vi "Read Data.vi"(8 "error in (no error)":errorcluster, 11 "Serial Config":T1={"串口选择"="", "通讯速率"=9600, "超时时间"=10000, "数据位长"=8, "奇偶校验"=enum."None", "停止位长"=10, "握手控制"=0, "字符结束"=TRUE, "结束字符"=10} {"结束字符" format="%.0x"; "握手控制" items=["None", "XON/XOFF", "RTS/CTS", "XON/XOFF & RTS/CTS", "DTR/DSR", "XON/XOFF & DTR/DSR"]; "停止位长" items=["1.0"=10, "1.5"=15, "2.0"=20]; "数据位长" min=5 max=8 step=1}) -> (0 "error out":errorcluster, 2 "状态信息":string, 3 "返回值":dbl)   [LabVIEW 2010, in "CenterOne.lvlib"]
doc: "Use this template to build a VI to use as a subVI."
uses:
  CenterOne.lvlib
  Serial Config.ctl
  <vilib>/Instr/_visa.llb/VISA Configure Serial Port (Instr).vi
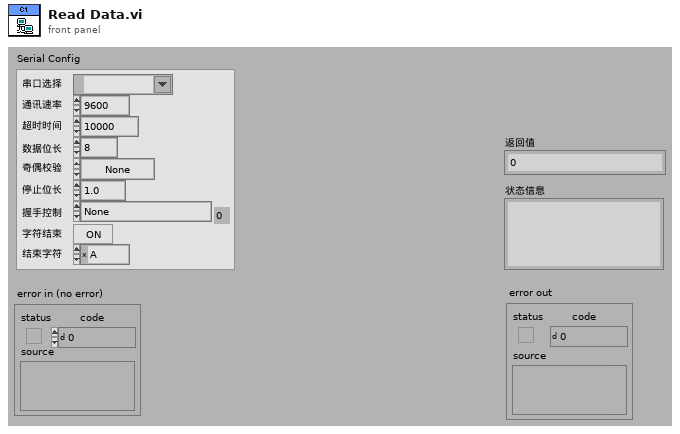
[diagram p1: front panel]
types:
  T1 = typedef "CenterOne.lvlib/Serial Config.ctl" = cluster{"串口选择":refnum<visa-resource-name>, "通讯速率":u32, "超时时间":u32, "数据位长":u16, "奇偶校验":enum16{"None", "Odd", "Even", "Mark", "Space"}, "停止位长":u16, "握手控制":u16, "字符结束":bool, "结束字符":u8}
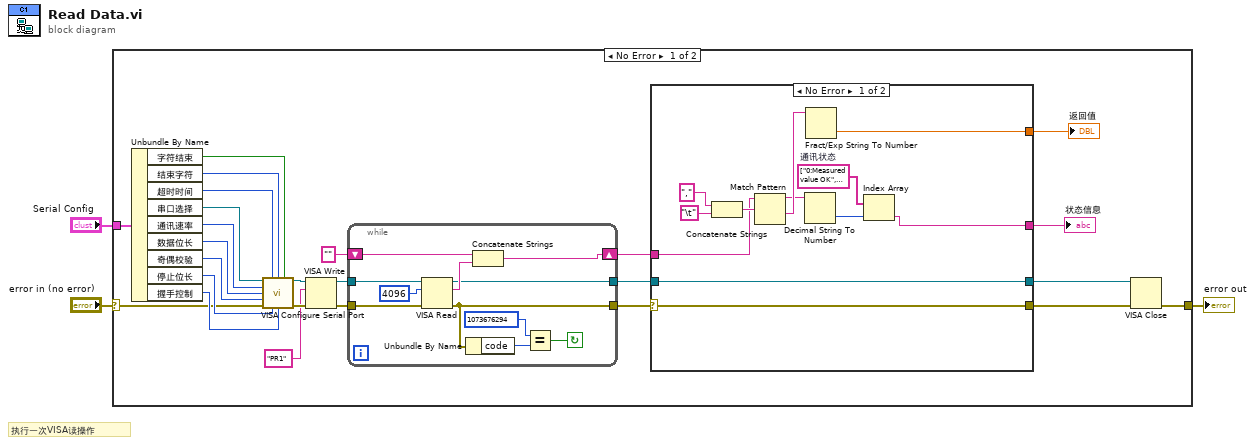
[diagram p0: block diagram]
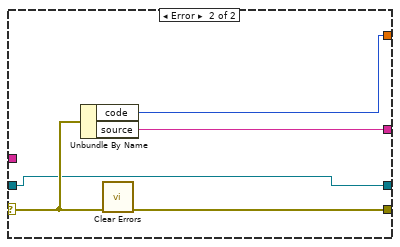
[diagram p2: hidden frame]
diagram:
  # "执行一次VISA读操作"
  n1 = case shown="No Error" "error in (no error)" {
    selector: "error in (no error)" -> [w16 w57]
    tunnel: [w15 w57] -> w2
    tunnel: "Serial Config" -> [w26 _]
    frame No Error {
      n2 = Unbundle By Name(w26) -> ("字符结束"=w21:bool, "结束字符"=w22:u8, "超时时间"=w23:u32, "串口选择"=w25:refnum<visa-resource-name>, "通讯速率"=w24:u32, "数据位长"=w20:u16, "奇偶校验"=w19:enum16{"None", "Odd", "Even", "Mark", "Space"}, "停止位长"=w18:u16, "握手控制"=w17:u16)
      n3 = call-poly "VISA Configure Serial Port"("VISA resource name"=w25, "timeout (10sec)"=w23, "termination char\n(0xA = '\\n' = LF)"=w22, "Enable Termination\nChar (T)"=w21, "baud rate (9600)"=w24, "data bits (8)"=w20, "parity (0:none)"=w19, "error in (no error)"=w16, "stop bits (10: 1 bit)"=w18, "flow control (0:none)"=w17) -> ("VISA resource name out"=w27:refnum<visa-resource-name>, "error out"=w28:errorcluster)  [unwired: 4 in]
      n4 = VISA Write(VISA resource name=w27, write buffer="PR1", error in (no error)=w28) -> (VISA resource name out=w13:refnum<visa-resource-name>, error out=w12:errorcluster)  [unwired: 1 out]
      n5 = while {
        shift-left: "" -> [w50]
        shift-right: [w49] -> w9
        tunnel: [w52] -> w8
        tunnel: w13 -> [w48]
        tunnel: w12 -> [w47]
        tunnel: [w46] -> w6
        stop <- w54 continue-if-true
        n6 = VISA Read(VISA resource name=w48, byte count=u32 4096 ("byte count (0)"), error in (no error)=w47) -> (VISA resource name out=w46:refnum<visa-resource-name>, read buffer=w51:string, error out=w52:errorcluster)  [unwired: 1 out]
        n7 = Unbundle By Name(w52) -> ("code"=w55:i32)
        n8 = Concatenate Strings(w50, w51) -> (w49:string)
        n9 = Equal?(x=1073676294, y=w55) -> (x = y?=w54:bool)
      }
      n10 = case shown="No Error" w8 {
        selector: w8 -> [w30 w44]
        tunnel: [w30 w45] -> w10
        tunnel: w9 -> [w33 _]
        tunnel: [w32 w43] -> w7
        tunnel: w6 -> [w31 w42]
        tunnel: [w31 w42] -> w5
        tunnel: [w29 w41] -> w4
        frame No Error {
          w39 = string[] ["0:Measured value OK", "1:Measured value < measurement range", "2:Measured value > measurement range", "3:Measured values significantly < measurement range(Err Lo)", "4:Measured values significantly > measurement range(Err Hi)", "5:Sensor off (S oFF)", "6:HV on (HU on)", "7:Sensor error (Err S)", "8:No Define", "9:No sensor(no Sen)", "10:No switch-on or switch-off threshold (notriG)", "11:No Define", "12:Pirani error (Err Pi)", "\n"]  # 通讯状态
          n11 = Concatenate Strings("," ("正则表达式"), "\t") -> (w36:string)
          n12 = Match Pattern(string=w33, regular expression=w36) -> (before substring=w37:string, after substring=w38:string)  [unwired: 1 in, 2 out]
          n13 = Decimal String To Number(string=w37) -> (number=w40:i32)  [unwired: 2 in, 1 out]
          n14 = Fract/Exp String To Number(string=w38) -> (number=w29:dbl)  [unwired: 3 in, 1 out]
          n15 = Index Array(array=w39, index=w40) -> (element=w32:string)
        }
        frame Error {
          n16 = Unbundle By Name(w44) -> ("code"=w41:i32, "source"=w43:string)
          n17 = call <vilib>:"Clear Errors.vi"("error in (no error)"=w44) -> ("error out"=w45:errorcluster)  [unwired: 6 in]
        }
      }
      "状态信息" <- w7
      "返回值" <- w4
      n18 = VISA Close(VISA resource name=w5, error in (no error)=w10) -> (error out=w15:errorcluster)
    }
    frame Error {
    }
  }
  "error out" <- w2
